vi "High_Power_CH2.vi"(8 "Modulation parameter":T1, 9 "output bits":i8[](array[numeric]), 10 "Boolean":bool, 11 "Record BER":bool) -> ()   [LabVIEW 2022 SP3]
panel:
  out "No. Bits LP":dbl
  out "?":T1
  out "Low-Power Decoded Message":string
  in  "Expected message LP":string="Non Critical Data\nNon Critical Data\nNon Critical Data\nNon Critical Data\nNon Critical Data"
  out "Acum. Err LP":dbl
  out "Acc. BER LP":dbl format="%#_4g"
  out "Inst. BER LP":dbl format="%#_4g"
  out "Low-Power BER Graph":dbl(graph)
  out "Low-Power Instantaneous BER Graph":u8(slide) scale=0.0..100.0
  in  "Low-Power Window Size":dbl=15.0 format="%#_6p"
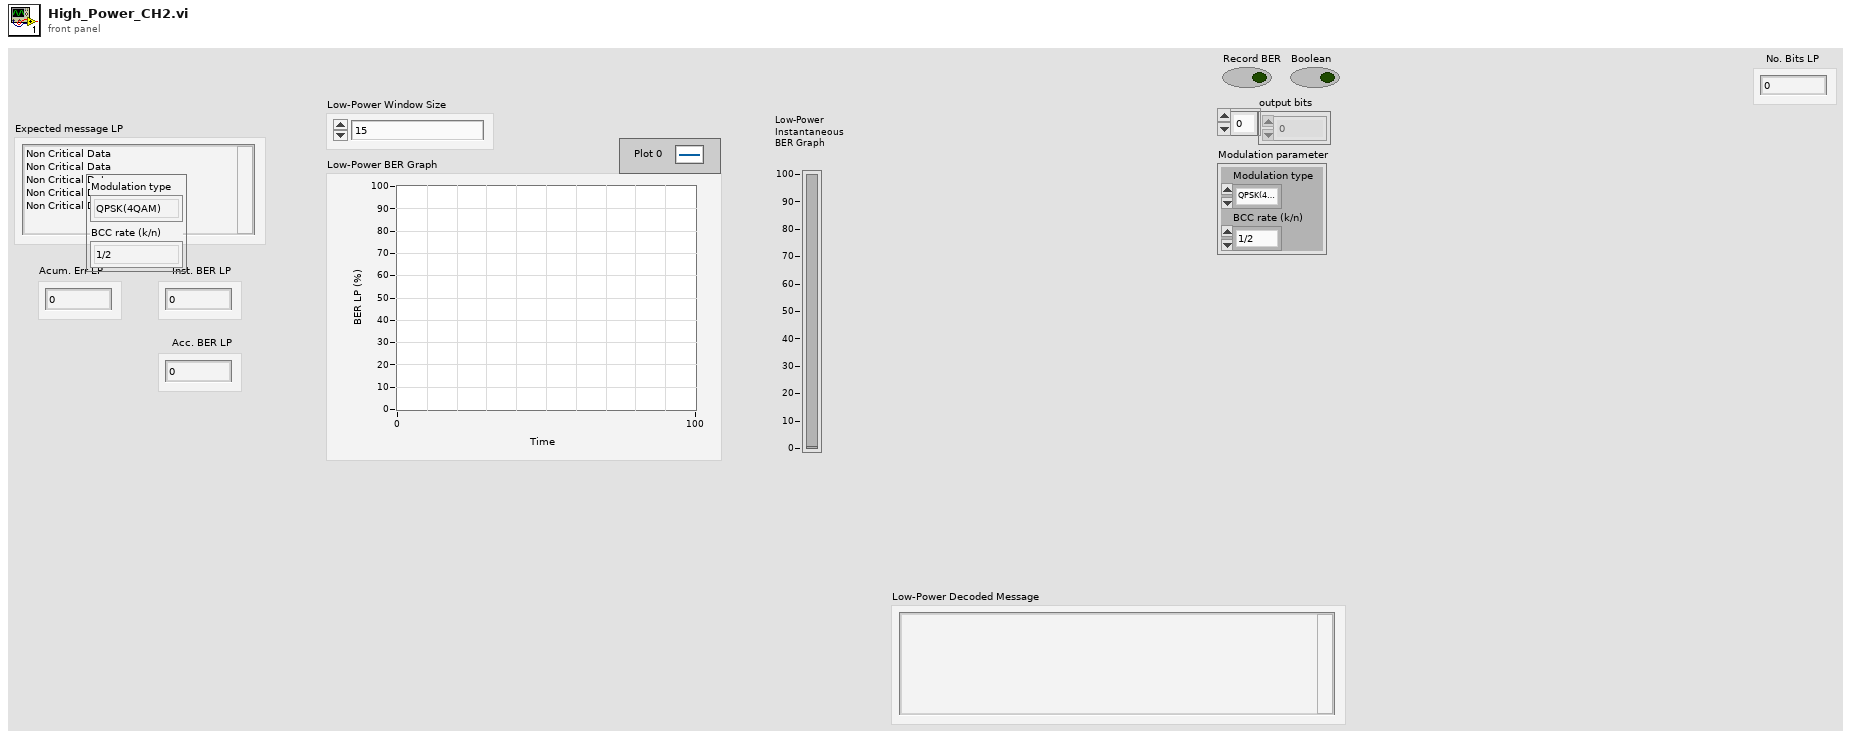
[diagram p1: front panel]
types:
  T1 = cluster{"Modulation type":enum16{"QPSK(4QAM)", "64QAM", "16QAM", "BPSK"}, "BCC rate (k/n)":enum16{"1/2", "2/3", "3/4"}}
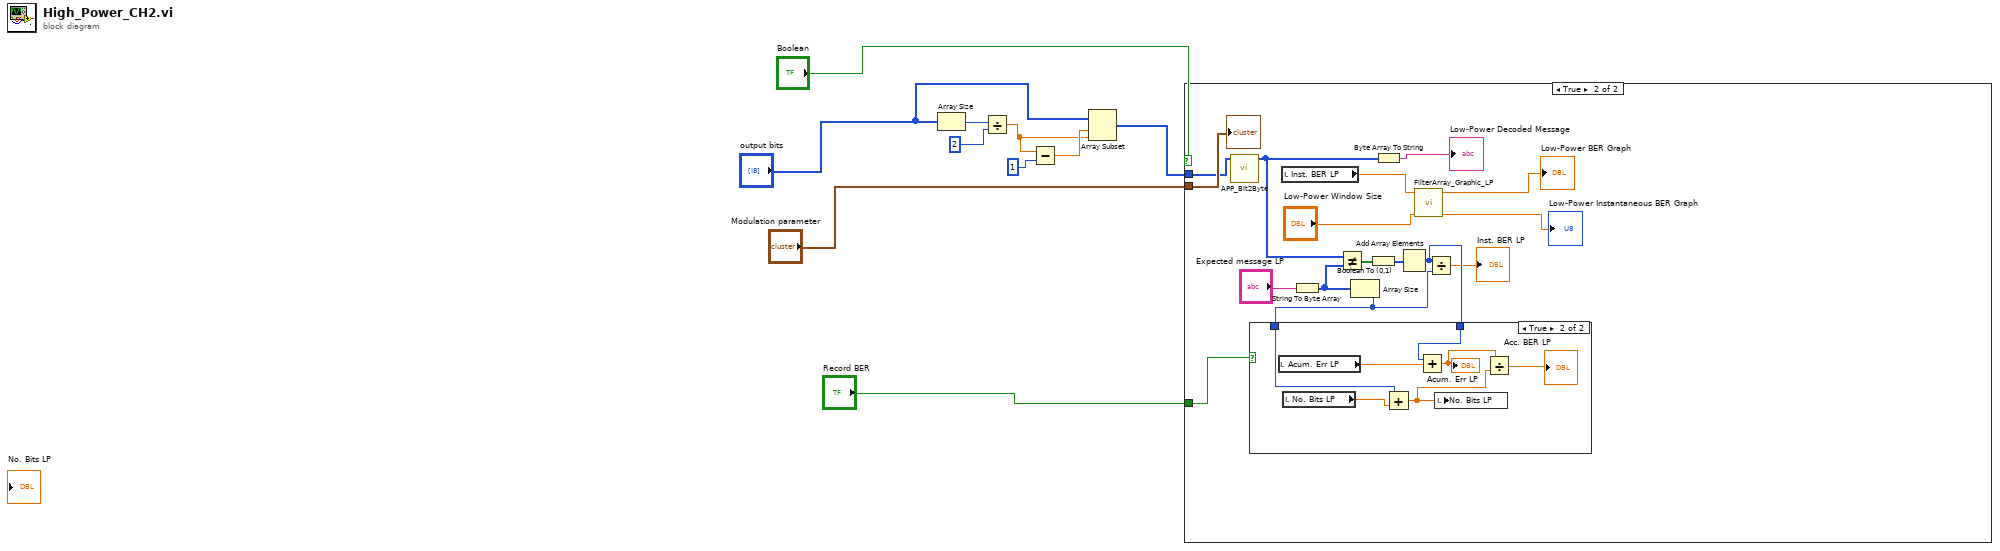
[diagram p0: block diagram]
diagram:
  n1 = Array Size(array="output bits") -> (size(s)=w7:i32)
  n2 = Divide(x=w7, y=2) -> (x/y=w2:dbl)
  n3 = Subtract(x=w2, y=1) -> (x-y=w3:dbl)
  n4 = Array Subset(array="output bits", index=w3, length=w2) -> (w1:i8[])
  n5 = case shown="True" "Boolean" {
    tunnel: "Modulation parameter" -> [_ w26]
    tunnel: "Record BER" -> [_ w17]
    tunnel: w1 -> [_ w11]
    frame False {
    }
    frame True {
      n6 = call "APP_Bit2Byte.vi"("input bit stream"=w11) -> ("output byte stream"=w19:u8[])  [unwired: 10 in]
      n7 = local read "Inst. BER LP"() -> (w15:dbl)
      n8 = String To Byte Array(string="Expected message LP") -> (unsigned byte array=w23:u8[])
      n9 = Not Equal?(x=w19, y=w23) -> (x != y?=w21:bool[])
      n10 = Array Size(array=w23) -> (size(s)=w24:i32)
      n11 = Boolean To (0,1)(Boolean=w21) -> (0, 1=w20:i16[])
      n12 = Byte Array To String(unsigned byte array=w19) -> (string=→"Low-Power Decoded Message":string)
      n13 = Add Array Elements(numeric array=w20) -> (sum=w18:i16)
      n14 = case shown="True" w17 {
        tunnel: w24 -> [_ w32]
        tunnel: w18 -> [_ w30]
        frame False {
        }
        frame True {
          n15 = local read "Acum. Err LP"() -> (w31:dbl)
          n16 = local read "No. Bits LP"() -> (w33:dbl)
          n17 = Add(x=w32, y=w33) -> (x+y=w27:dbl)
          n18 = Add(x=w30, y=w31) -> (x+y=w29:dbl)
          "Acum. Err LP" <- w29
          n19 = local write "No. Bits LP"(w27) -> ()
          n20 = Divide(x=w29, y=w27) -> (x/y=→"Acc. BER LP":dbl)
        }
      }
      n21 = call "FilterArray_Graphic_LP.vi"("Window Size"="Low-Power Window Size", "Instantaneous BER"=w15) -> ("Slide Bar"=→"Low-Power Instantaneous BER Graph":dbl, "Graph Instantaneous BER"=→"Low-Power BER Graph":dbl)  [unwired: 4 in]
      n22 = Divide(x=w18, y=w24) -> (x/y=→"Inst. BER LP":dbl)
      "?" <- w26
    }
  }
